vi "Write Snapshot.vi"(8 "error in (no error)":errorcluster, 10 "Snapshot":waveform(dbl)[](array[waveform]), 11 "Instruments in":refnum<class "Instruments.lvclass">) -> (0 "error out":errorcluster, 3 "Instruments out":refnum<class "Instruments.lvclass">)   [LabVIEW 2023, in "Instruments.lvlib" / "Instruments.lvclass"]
uses:
  Library/Instruments.lvclass
  Library/Instruments.lvclass/Instruments.ctl
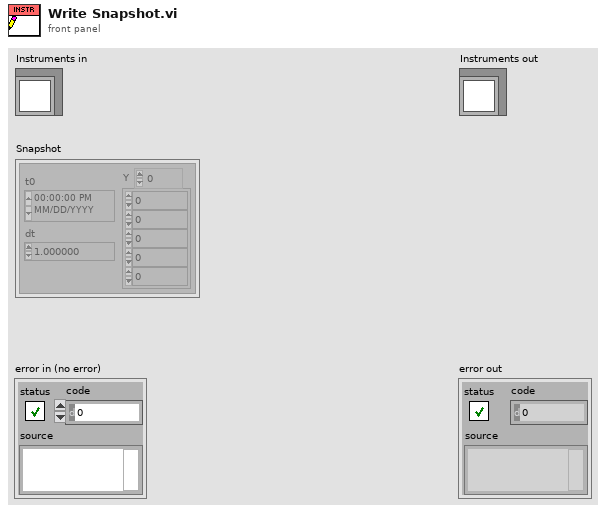
[diagram p1: front panel]
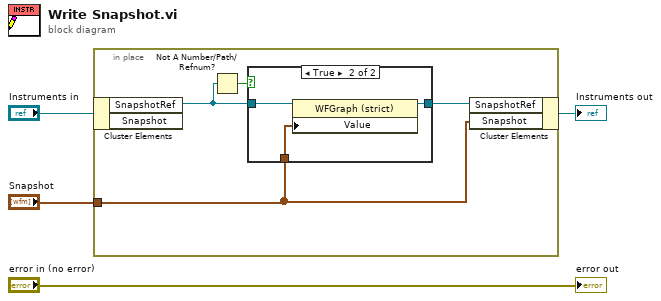
[diagram p0: block diagram]
diagram:
  n1 = in-place {
    in-place-border: "Snapshot" -> [w7]
    n2 = in-place-cluster #1("Instruments in") -> ("SnapshotRef"=w5:refnum<vi>)  [unwired: 1 out]
    n3 = Not A Number/Path/Refnum?(number/path/refnum=w5) -> (NaN/Path/Refnum?=w6:bool)
    n4 = case shown="True" w6 {
      tunnel: w5 -> [w9 w12]
      tunnel: [w9 w11] -> w8
      tunnel: w7 -> [_ w10]
      frame False {
      }
      frame True {
        n5 = property class="WFGraph (strict)"(reference=w12, "Value"=w10) -> (reference out=w11:refnum<vi>)  [unwired: 1 in, 1 out]
      }
    }
    n6 = in-place-cluster #1("SnapshotRef"=w8, "Snapshot"=w7) -> (→"Instruments out":refnum<class "Instruments.lvclass">)
  }
  "error out" <- "error in (no error)"
